vi "Tree.vi"() -> ()   [LabVIEW 2016]
uses:
  Data/Data.lvclass
  Data.ITX/Data.ITX.lvclass
  Data.DAT/Data.DAT.lvclass
  Data.TDMS/Data.TDMS.lvclass
  Macros/Conversion.lvclass
  Data.HDF5/Data.HDF5.lvclass
  Data.DAT/Write DAT (1D).vi
  Data/API/XY-Data to Dictionary (single).vi
  Data/API/XY-Data to Dictionary (Multiple).vi
  Data/Typedefs/File Type--enum.ctl
  Data/Typedefs/Operation--enum.ctl
  Data/Typedefs/Dictionary--cluster.ctl
panel:
  in  "Append Index":i32
  in  "File Type":T1
  in  "error in (no error)":errorcluster
  in  "Notes":string
  in  "Data (Dictionary)":T2[](array[typedef])
  in  "path":path
  out "path out":path
  out "Data (Dictionary) out":T2[](array[typedef])
  out "Notes out":string
  out "error out":errorcluster
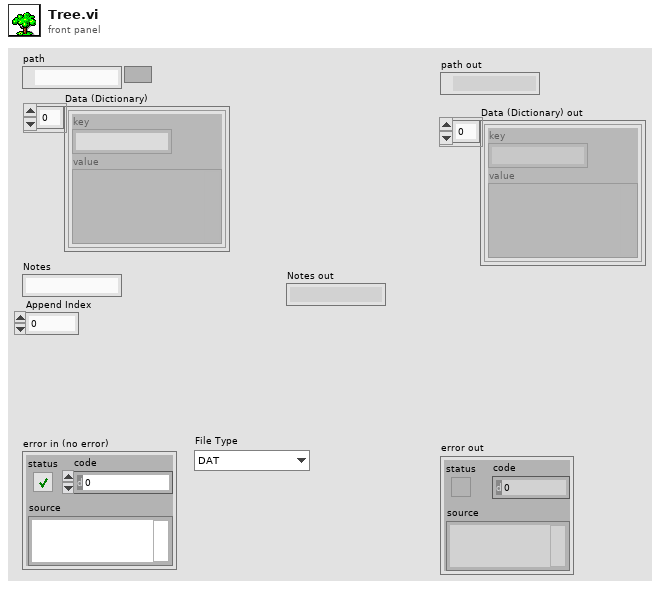
[diagram p1: front panel]
types:
  T1 = typedef "Data.lvclass/File Type--enum.ctl" = enum16{"DAT", "ITX", "HDF5", "TDMS", "VI", "PGSQL"}
  T2 = typedef "Data.lvclass/Dictionary--cluster.ctl" = cluster{"key":string, "value":variant}
  T3 = typedef "Data.lvclass/Operation--enum.ctl" = enum16{"Read", "Write", "Write + Append"}
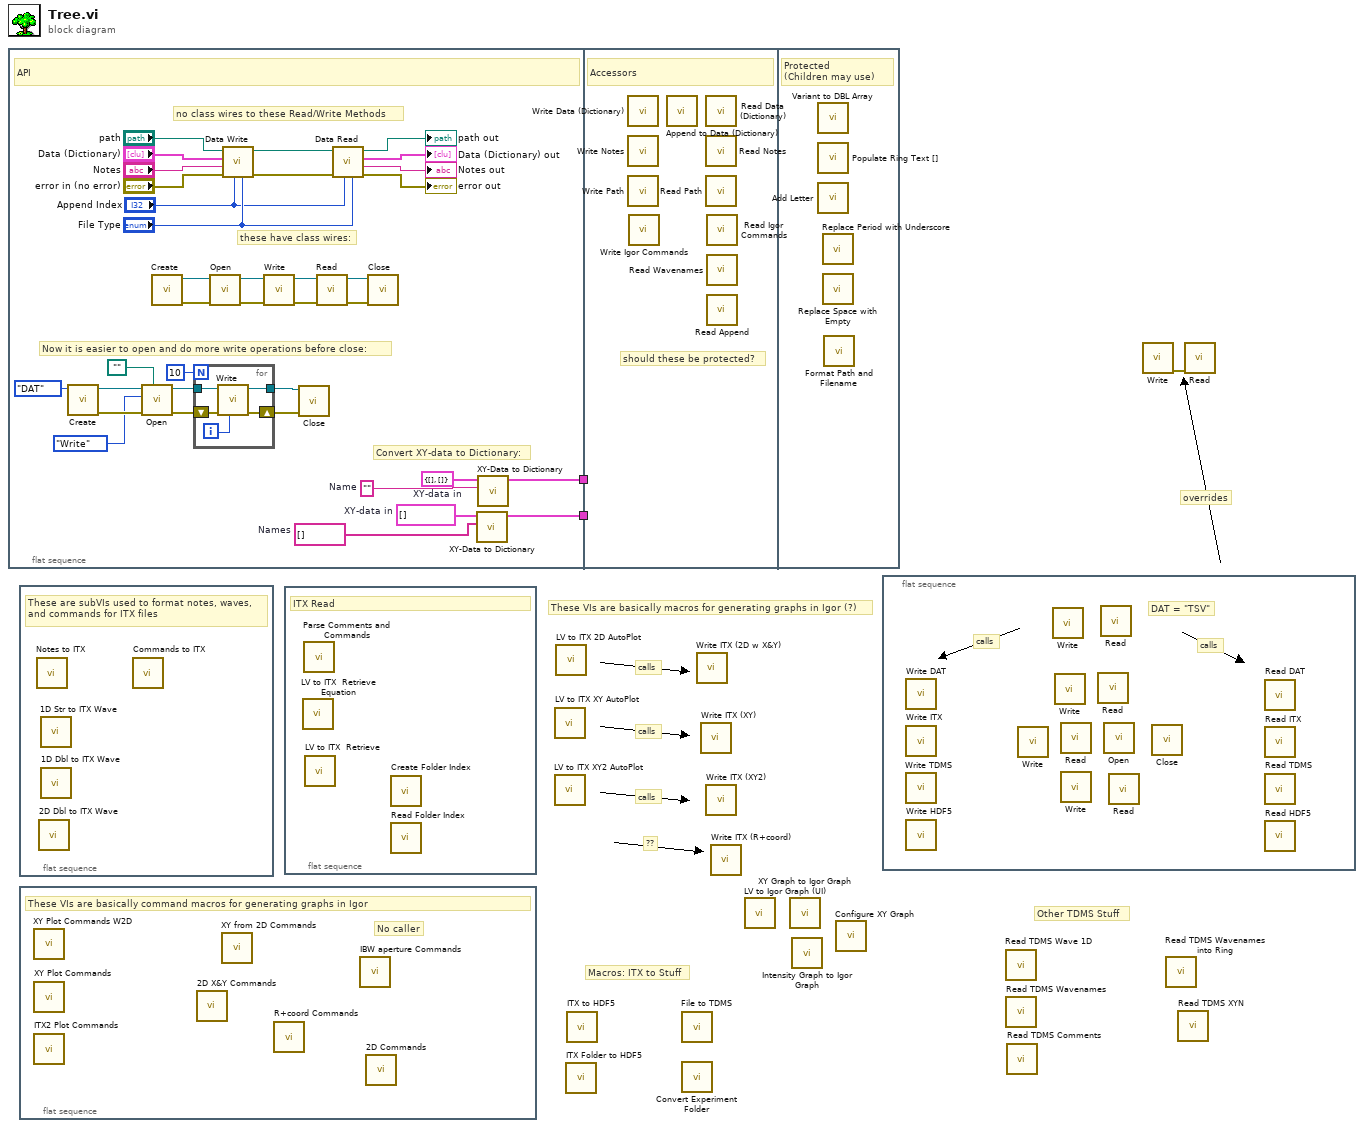
[diagram p0: block diagram]
diagram:
  # "??"
  # "calls"
  # "calls"
  # "calls"
  # "overrides"
  # "Macros: ITX to Stuff"
  # "Other TDMS Stuff"
  # "These VIs are basically macros for generating graphs in Igor (?)"
  n1 = flat-sequence {
    tunnel: [w31] -> w3
    tunnel: [w29] -> w2
    tunnel: w3 -> [_]
    tunnel: w2 -> [_]
    frame #0 {
      w27 = string[] []  # Names
      w28 = ""  # Name
      w30 = cluster{"X-array":dbl[], "Y-array":dbl[]}[] []  # XY-data in
      w32 = cluster{"X-array":dbl[], "Y-array":dbl[]} {"X-array"=[], "Y-array"=[]}  # XY-data in
      # "Now it is easier to open and do more write operations before close:"
      # "Convert XY-data to Dictionary:"
      # "these have class wires:"
      # "no class wires to these Read/Write Methods"
      # "API"
      n2 = call "Create.vi"("File Type"=File_Type--enum."DAT") -> ("error out"=w18:errorcluster, "Data out"=w17:refnum<class "Data.lvclass">)  [unwired: 9 in]
      n3 = call-dynamic "Open.vi"("Path"=path "", "error in (no error)"=w18, "Operation"=Operation--enum."Write", "Data in"=w17) -> ("error out"=w16:errorcluster, "Data out"=w15:refnum<class "Data.lvclass">)  [unwired: 6 in]
      n4 = call "Create.vi"() -> ("error out"=w25:errorcluster, "Data out"=w26:refnum<class "Data.lvclass">)  [unwired: 10 in]
      n5 = for {
        N: 10 -> [_]
        tunnel: w15 -> [w42]
        tunnel: [w40] -> w13
        shift-right: [w41] -> w14
        shift-left: w16 -> [w43]
        i -> [w44]
        n6 = call-dynamic "Write.vi"("Append Index"=w44, "error in (no error)"=w43, "Data in"=w42) -> ("error out"=w41:errorcluster, "Data out"=w40:refnum<class "Data.lvclass">)  [unwired: 6 in, 1 out]
      }
      n7 = call-dynamic "Open.vi"("error in (no error)"=w25, "Data in"=w26) -> ("error out"=w23:errorcluster, "Data out"=w24:refnum<class "Data.lvclass">)  [unwired: 8 in]
      n8 = call "Data Write.vi"("File Type"="File Type", "Append Index"="Append Index", "error in (no error)"="error in (no error)", "Notes"="Notes", "Data (Dictionary)"="Data (Dictionary)", "path"="path") -> ("error out"=w38:errorcluster, "path out"=w9:path)  [unwired: 4 in]
      n9 = call-dynamic "Write.vi"("error in (no error)"=w23, "Data in"=w24) -> ("error out"=w21:errorcluster, "Data out"=w22:refnum<class "Data.lvclass">)  [unwired: 7 in, 1 out]
      n10 = call-dynamic "Close.vi"("error in (no error)"=w14, "Data in"=w13) -> ()  [unwired: 8 in, 2 out]
      n11 = call-dynamic "Read.vi"("error in (no error)"=w21, "Data Save in"=w22) -> ("error out"=w19:errorcluster, "Data Save out"=w20:refnum<class "Data.lvclass">)  [unwired: 5 in, 3 out]
      n12 = call "Data Read.vi"(4:"File Type", "Append Index"="Append Index", "error in (no error)"=w38, "path"=w9) -> ("error out"=→"error out":errorcluster, "Notes"=→"Notes out":string, "Data (Dictionary)"=→"Data (Dictionary) out":T2[], "path out"=→"path out":path)  [unwired: 4 in]
      n13 = call-dynamic "Close.vi"("error in (no error)"=w19, "Data in"=w20) -> ()  [unwired: 8 in, 2 out]
      n14 = call-poly "XY-Data to Dictionary.vi"("Names"=w27, "XY-data in"=w30) -> ("Data (Dictionary)"=w29:T2[])  [unwired: 8 in, 1 out]
      n15 = call-poly "XY-Data to Dictionary.vi"("Name"=w28, "XY-data in"=w32) -> ("Data (Dictionary)"=w31:T2[])  [unwired: 8 in, 1 out]
    }
    frame #1 {
      # "should these be protected?"
      # "Accessors"
      n16 = call "Write Data (Dictionary).vi"() -> ()  [unwired: 10 in, 2 out]
      n17 = call "Write Notes.vi"() -> ()  [unwired: 10 in, 2 out]
      n18 = call "Write Path.vi"() -> ()  [unwired: 10 in, 2 out]
      n19 = call "Write Igor Commands.vi"() -> ()  [unwired: 10 in, 2 out]
      n20 = call "Append to Data (Dictionary).vi"() -> ()  [unwired: 10 in, 2 out]
      n21 = call "Read Data (Dictionary).vi"() -> ()  [unwired: 9 in, 3 out]
      n22 = call "Read Notes.vi"() -> ()  [unwired: 9 in, 3 out]
      n23 = call "Read Path.vi"() -> ()  [unwired: 9 in, 3 out]
      n24 = call "Read Igor Commands.vi"() -> ()  [unwired: 9 in, 3 out]
      n25 = call "Read Wavenames.vi"() -> ()  [unwired: 9 in, 3 out]
      n26 = call "Read Append.vi"() -> ()  [unwired: 9 in, 3 out]
    }
    frame #2 {
      # "Protected\n(Children may use)"
      n27 = call "Variant to DBL Array.vi"() -> ()  [unwired: 9 in, 3 out]
      n28 = call "Populate Ring Text [].vi"() -> ()  [unwired: 11 in, 1 out]
      n29 = call "Add Letter.vi"() -> ()  [unwired: 1 in, 1 out]
      n30 = call "Replace Period with Underscore.vi"() -> ()  [unwired: 1 in, 1 out]
      n31 = call "Replace Space with Empty.vi"() -> ()  [unwired: 1 in, 1 out]
      n32 = call "Format Path and Filename.vi"() -> ()  [unwired: 10 in, 2 out]
    }
  }
  n33 = flat-sequence {
    frame #0 {
      # "These are subVIs used to format notes, waves, and commands for ITX files"
      n34 = call "Notes to ITX.vi"() -> ()  [unwired: 1 in, 1 out]
      n35 = call "2D Dbl to ITX Wave.vi"() -> ()  [unwired: 2 in, 1 out]
      n36 = call "1D Str to ITX Wave.vi"() -> ()  [unwired: 2 in, 1 out]
      n37 = call "1D Dbl to ITX Wave.vi"() -> ()  [unwired: 2 in, 1 out]
      n38 = call "Commands to ITX.vi"() -> ()  [unwired: 1 in, 1 out]
    }
  }
  n39 = flat-sequence {
    frame #0 {
      # "No caller"
      # "These VIs are basically command macros for generating graphs in Igor"
      n40 = call "XY Plot Commands W2D.vi"() -> ()  [unwired: 5 in, 1 out]
      n41 = call "XY Plot Commands.vi"() -> ()  [unwired: 6 in, 1 out]
      n42 = call "ITX2 Plot Commands.vi"() -> ()  [unwired: 6 in, 1 out]
      n43 = call "2D X&Y Commands.vi"() -> ()  [unwired: 10 in, 2 out]
      n44 = call "XY from 2D Commands.vi"() -> ()  [unwired: 2 in, 1 out]
      n45 = call "R+coord Commands.vi"() -> ()  [unwired: 15 in, 1 out]
      n46 = call "IBW aperture Commands.vi"() -> ()  [unwired: 4 in, 1 out]
      n47 = call "2D Commands.vi"() -> ()  [unwired: 15 in, 1 out]
    }
  }
  n48 = flat-sequence {
    frame #0 {
      # "ITX Read"
      n49 = call "LV to ITX  Retrieve Equation.vi"() -> ()  [unwired: 11 in, 5 out]
      n50 = call "Parse Comments and Commands.vi"() -> ()  [unwired: 2 in, 2 out]
      n51 = call "LV to ITX  Retrieve.vi"() -> ()  [unwired: 11 in, 5 out]
      n52 = call "Create Folder Index.vi"() -> ()  [unwired: 11 in, 1 out]
      n53 = call "Read Folder Index.vi"() -> ()  [unwired: 10 in, 2 out]
    }
  }
  n54 = call "LV to ITX XY AutoPlot.vi"() -> ()  [unwired: 10 in, 2 out]
  n55 = call "LV to ITX XY2 AutoPlot.vi"() -> ()  [unwired: 10 in, 2 out]
  n56 = call "LV to ITX 2D AutoPlot.vi"() -> ()  [unwired: 10 in, 2 out]
  n57 = call "ITX Folder to HDF5.vi"() -> ()  [unwired: 11 in, 1 out]
  n58 = call "ITX to HDF5.vi"() -> ()  [unwired: 11 in, 1 out]
  n59 = call "File to TDMS.vi"() -> ()  [unwired: 9 in, 3 out]
  n60 = call "Convert Experiment Folder.vi"() -> ()  [unwired: 11 in, 1 out]
  n61 = call "Write ITX (2D w X&Y).vi"() -> ()  [unwired: 10 in, 2 out]
  n62 = call "Write ITX (XY).vi"() -> ()  [unwired: 10 in, 2 out]
  n63 = call "Write ITX (XY2).vi"() -> ()  [unwired: 10 in, 2 out]
  n64 = call "Write ITX (R+coord).vi"() -> ()  [unwired: 12 in]
  n65 = call "LV to Igor Graph (UI).vi"() -> ()  [unwired: 12 in]
  n66 = call "XY Graph to Igor Graph.vi"() -> ()  [unwired: 10 in, 2 out]
  n67 = call "Intensity Graph to Igor Graph.vi"() -> ()  [unwired: 10 in, 2 out]
  n68 = call "Configure XY Graph.vi"() -> ()  [unwired: 11 in, 1 out]
  n69 = flat-sequence {
    frame #0 {
      # "DAT = \"TSV\""
      # "calls"
      # "calls"
      n70 = call-poly "Write DAT.vi"() -> ()  [unwired: 10 in, 2 out]
      n71 = call "Write ITX.vi"() -> ()  [unwired: 10 in, 2 out]
      n72 = call "Write TDMS.vi"() -> ()  [unwired: 10 in, 2 out]
      n73 = call "Write HDF5.vi"() -> ()  [unwired: 10 in, 2 out]
      n74 = call-dynamic "Write.vi"() -> ()  [unwired: 9 in, 3 out]
      n75 = call-dynamic "Write.vi"() -> ()  [unwired: 9 in, 3 out]
      n76 = call-dynamic "Write.vi"() -> ()  [unwired: 9 in, 3 out]
      n77 = call-dynamic "Read.vi"() -> ()  [unwired: 7 in, 5 out]
      n78 = call-dynamic "Write.vi"() -> ()  [unwired: 9 in, 3 out]
      n79 = call-dynamic "Read.vi"() -> ()  [unwired: 7 in, 5 out]
      n80 = call-dynamic "Read.vi"() -> ()  [unwired: 7 in, 5 out]
      n81 = call-dynamic "Open.vi"() -> ()  [unwired: 10 in, 2 out]
      n82 = call-dynamic "Read.vi"() -> ()  [unwired: 7 in, 5 out]
      n83 = call-dynamic "Close.vi"() -> ()  [unwired: 10 in, 2 out]
      n84 = call "Read DAT.vi"() -> ()  [unwired: 9 in, 3 out]
      n85 = call "Read ITX.vi"() -> ()  [unwired: 8 in, 4 out]
      n86 = call "Read TDMS.vi"() -> ()  [unwired: 8 in, 4 out]
      n87 = call "Read HDF5.vi"() -> ()  [unwired: 8 in, 4 out]
    }
  }
  n88 = call "Read TDMS Wave 1D.vi"() -> ()  [unwired: 9 in, 3 out]
  n89 = call "Read TDMS Wavenames.vi"() -> ()  [unwired: 9 in, 3 out]
  n90 = call "Read TDMS Comments.vi"() -> ()  [unwired: 10 in, 2 out]
  n91 = call-dynamic "Write.vi"() -> ("error out"=w1:errorcluster)  [unwired: 9 in, 2 out]
  n92 = call "Read TDMS Wavenames into Ring.vi"() -> ()  [unwired: 11 in, 1 out]
  n93 = call "Read TDMS XYN.vi"() -> ()  [unwired: 9 in, 3 out]
  n94 = call-dynamic "Read.vi"("error in (no error)"=w1) -> ()  [unwired: 6 in, 5 out]
